vi "Process Data Conifg PID Gain_vel.vi"(8 "에러 입력(에러 없음)":errorcluster) -> (0 "에러 출력":errorcluster, 3 "출력 클러스터":T1)   [LabVIEW 2019]
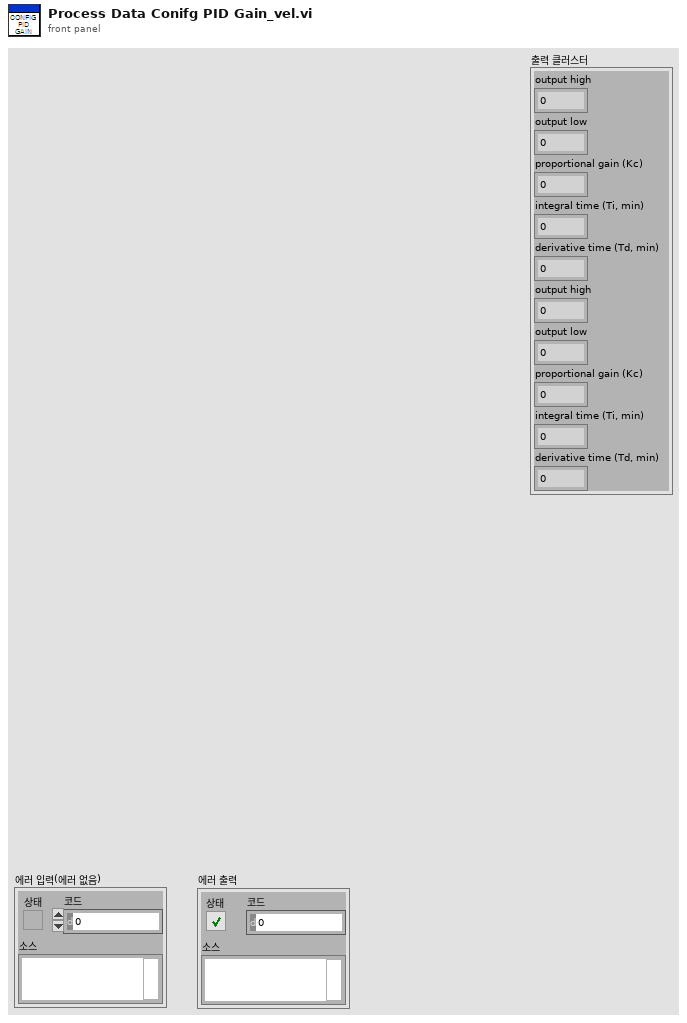
[diagram p1: front panel]
types:
  T1 = cluster{"output high":dbl, "output low":dbl, "proportional gain (Kc)":dbl, "integral time (Ti, min)":dbl, "derivative time (Td, min)":dbl, "output high":dbl, "output low":dbl, "proportional gain (Kc)":dbl, "integral time (Ti, min)":dbl, "derivative time (Td, min)":dbl}
  T2 = enum16{"open", "replace", "create", "open or create", "replace or create", "replace or create with confirmation"}
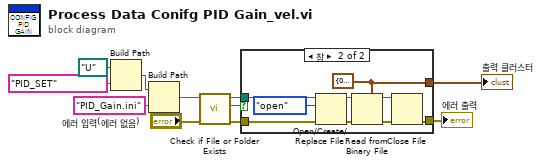
[diagram p0: block diagram]
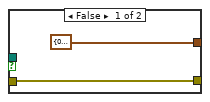
[diagram p2: hidden frame]
diagram:
  n1 = Build Path(base path=path "U:/" ("베이스 경로"), name or relative path="PID_SET" ("시간 포맷 문자열 (%c)")) -> (appended path=w5:path)
  n2 = Build Path(base path=w5, name or relative path="PID_Gain.ini" ("이름 또는 상대 경로")) -> (appended path=w6:path)
  n3 = call <vilib>:"Check if File or Folder Exists.vi"("error in (no error)"="에러 입력(에러 없음)", "path"=w6) -> ("error out"=w9:errorcluster, "file or folder exists?"=w7:bool, "dup path"=w8:path)  [unwired: 7 in]
  n4 = case shown="참" w7 {
    tunnel: w8 -> [_ w18]
    tunnel: w9 -> [w13 w17]
    tunnel: [T1 {"output high"=0.0, "output low"=0.0, "proportional gain (Kc)"=0.0, "integral time (Ti, min)"=0.0, "derivative time (Td, min)"=0.0, "output high"=0.0, "output low"=0.0, "proportional gain (Kc)"=0.0, "integral time (Ti, min)"=0.0, "derivative time (Td, min)"=0.0} ("출력 클러스터") w14] -> w1
    tunnel: [w13 w15] -> w11
    frame False {
    }
    frame True {
      w14 = T1 {"output high"=0.0, "output low"=0.0, "proportional gain (Kc)"=0.0, "integral time (Ti, min)"=0.0, "derivative time (Td, min)"=0.0, "output high"=0.0, "output low"=0.0, "proportional gain (Kc)"=0.0, "integral time (Ti, min)"=0.0, "derivative time (Td, min)"=0.0} ("출력 클러스터")
      n5 = Open/Create/Replace File(file path (use dialog)=w18, error in=w17, operation (0:open)=T2."open" ("동작(0:open)")) -> (refnum out=w21:refnum<file>, error out=w20:errorcluster)  [unwired: 3 in, 1 out]
      n6 = Read from Binary File(5:w14, 8:w20, 11:w21) -> (0:w16:errorcluster, 3:w19:refnum<file>)  [unwired: 3 in, 2 out]
      n7 = Close File(refnum=w19, error in=w16) -> (error out=w15:errorcluster)  [unwired: 1 out]
    }
  }
  "에러 출력" <- w11
  "출력 클러스터" <- w1
